vi "Filter Get Averaging Frame Count.vi"(11 "frames":i32) -> (2 "function return":u32, 3 "frames out":i32)   [LabVIEW 2018, in "AndorSDK.lvlib"]
doc: "EXPNETTYPE unsigned int WINAPI Filter_GetAveragingFrameCount(int * frames);"
uses:
  AndorSDK.lvlib
  ATMCD32D.dll
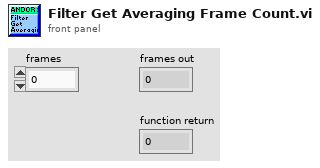
[diagram p1: front panel]
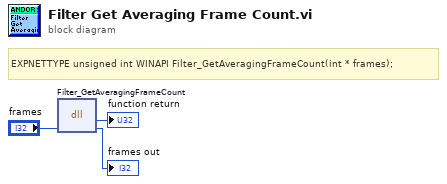
[diagram p0: block diagram]
diagram:
  # "EXPNETTYPE unsigned int WINAPI Filter_GetAveragingFrameCount(int * frames);"
  n1 = dll-call lib="PTH2babs E\nPersönliches02 - Arbeit03-HiwijobsLabviewCodelibANDOR\tAndor SDK\nATMCD32D.*" fn="Filter_GetAveragingFrameCount"("frames"="frames") -> (→"function return":u32, "frames"=→"frames out":i32)  [unwired: 3 in, 2 out]
